vi "DriveForDistance-C.vi"(11 "Params":string[][](array[string])) -> ()   [LabVIEW 2018]
uses:
  Framework/Robot Global Data.vi
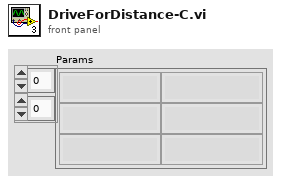
[diagram p1: front panel]
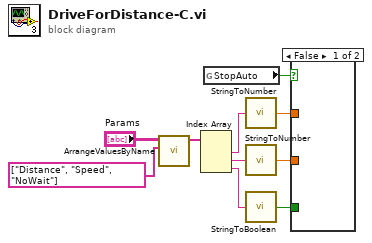
[diagram p0: block diagram]
diagram:
  n1 = call "ArrangeValuesByName.vi"("Names"=string[] ["Distance", "Speed", "NoWait"], "Names/Values in"="Params") -> ("Values Out"=w4:string[])  [unwired: 9 in]
  n2 = Index Array(array=w4) -> (element #1=w3:string, element #2=w2:string, element #3=w1:string)  [unwired: 3 in]
  n3 = global read "Robot Global Data.vi" "StopAuto"() -> (w7:bool)
  n4 = call "StringToNumber.vi"("String"=w3) -> ("Output"=w10:dbl)
  n5 = call "StringToNumber.vi"("String"=w2) -> ("Output"=w9:dbl)
  n6 = call "StringToBoolean.vi"("String"=w1) -> ("Output"=w8:bool)
  n7 = case shown="False" w7 {
    tunnel: w10 -> [_ _]
    tunnel: w9 -> [_ _]
    tunnel: w8 -> [_ _]
    frame False {
    }
    frame True {
    }
  }
